vi "rsscope Fetch Waveform.vi"(7 "Waveform (1)":i32=1, 8 "error in (no error)":errorcluster, 9 "Channel (1)":i32(ring)=1 items=["1"=1, "2"=2, "3"=3, "4"=4], 11 "VISA resource name":refnum<visa-resource-name>) -> (0 "error out":errorcluster, 2 "Waveform Array":dbl[](array[numeric]) format="%^.3e", 3 "VISA resource name out":refnum<visa-resource-name>, 4 "Initial X":dbl format="%^.3e", 5 "X Increment":dbl format="%^.3e")   [LabVIEW 2018]
doc: "This VI returns the waveform the oscilloscope acquires for the channel you specify. The waveform is from an acquisition that you previously initiated.\n\nYou use the rsscope Initiate Acquisition.vi to start an acquisition on the channels that you enable with the rsscope Configure Channel.vi. The oscilloscope acquires waveforms for the enabled channels concurrently. You use the rsscope_AcquisitionStatus VI to determine when the acquisition is complete. You must call this VI separately for each enabled channel to obtain the waveforms.\n\nYou can call the rsscope Read Waveform.vi instead of the rsscope Initiate Acquisition.vi. The rsscope Read Waveform.vi starts an acquisition on all enabled channels, waits for the acquisition to complete, and returns the waveform for the channel you specify. You call this VI to obtain the waveforms for each of the remaining channels.\n\nNotes:\n- After this VI executes, each element in the Waveform Array parameter is either a voltage or a value indicating that the oscilloscope could not sample a voltage.\n- You configure the interpolation method the oscilloscope uses with the rsscope Configure Interpolation.vi. If you disable interpolation, the oscilloscope does not interpolate points in the waveform.\n- This VI does not check the instrument status. Typically, you call this VI only in a sequence of calls to other low-level driver VIs. The sequence performs one operation. You use the low-level VIs to optimize one or more aspects of interaction with the instrument. If you want to check the instrument status, call the rsscope Error-Query.vi at the conclusion of the sequence.\n\nAttributes:\nRSSCOPE_ATTR_WAVEFORM_EXPORT_SCOPE_START\nRSSCOPE_ATTR_WAVEFORM_EXPORT_SCOPE_STOP\n\nRemote-control commands:\nEXPort:WAVeform:STARt\nEXPort:WAVeform:STOP\nCHANnel<m>[:WAVeform<n>]:DATA[:VALues]"
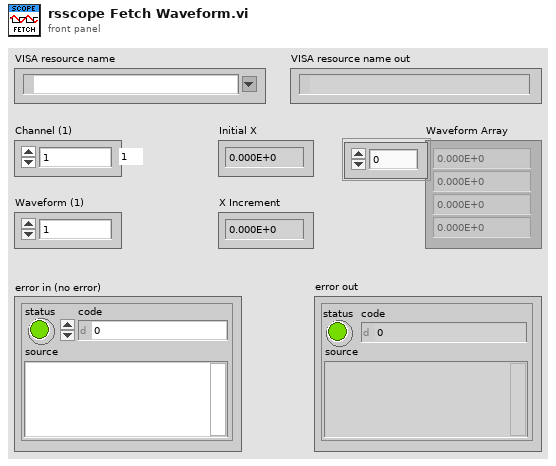
[diagram p1: front panel]
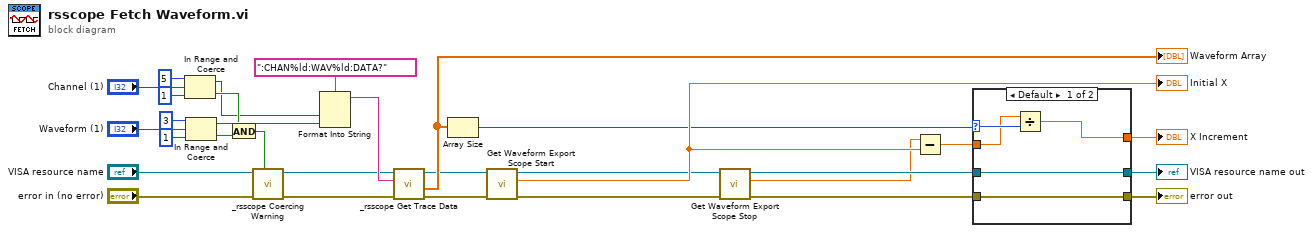
[diagram p0: block diagram]
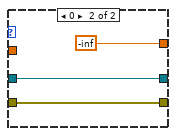
[diagram p2: hidden frame]
diagram:
  n1 = In Range and Coerce(upper limit=5, x="Channel (1)", lower limit=1) -> (coerced(x)=w2:i32, In Range?=w3:bool)
  n2 = In Range and Coerce(upper limit=3, x="Waveform (1)", lower limit=1) -> (coerced(x)=w5:i32, In Range?=w4:bool)
  n3 = And(x=w3, y=w4) -> (x .and. y?=w24:bool)
  n4 = call "_rsscope Coercing Warning.vi"("In Range?"=w24, "error in (no error)"="error in (no error)", "VISA resource name"="VISA resource name") -> ("error out"=w16:errorcluster, "VISA resource name out"=w15:refnum<visa-resource-name>)  [unwired: 7 in]
  n5 = Format Into String(format string=":CHAN%ld:WAV%ld:DATA?", w2, w5) -> (resulting string=w30:string)  [unwired: 2 in, 1 out]
  n6 = call "_rsscope Get Trace Data.vi"("error in (no error)"=w16, "Command"=w30, "VISA resource name"=w15) -> ("error out"=w14:errorcluster, "Values"=w19:dbl[], "VISA resource name out"=w13:refnum<visa-resource-name>)  [unwired: 6 in]
  "Waveform Array" <- w19
  n7 = Array Size(array=w19) -> (size(s)=w21:i32)
  n8 = call "Get Waveform Export Scope Start"("error in (no error)"=w14, "instrument handle"=w13) -> ("error out"=w9:errorcluster, "Waveform Export Scope Start"=w22:dbl, "instrument handle out"=w10:refnum<visa-resource-name>)  [unwired: 7 in]
  "Initial X" <- w22
  n9 = call "Get Waveform Export Scope Stop"("error in (no error)"=w9, "instrument handle"=w10) -> ("error out"=w7:errorcluster, "Waveform Export Scope Stop"=w1:dbl, "instrument handle out"=w8:refnum<visa-resource-name>)  [unwired: 7 in]
  n10 = Subtract(x=w1, y=w22) -> (x-y=w6:dbl)
  n11 = case shown="Default" w21 {
    selector: w21 -> [w36 _]
    tunnel: w8 -> [w32 w37]
    tunnel: [w32 w37] -> w11
    tunnel: w7 -> [w33 w39]
    tunnel: [w33 w39] -> w12
    tunnel: [w34 -inf ("X Increment")] -> w23
    tunnel: w6 -> [w35 _]
    frame Default {
      n12 = Divide(x=w35, y=w36) -> (x/y=w34:dbl)
    }
    frame 0 {
    }
  }
  "error out" <- w12
  "VISA resource name out" <- w11
  "X Increment" <- w23
